vi "Request Multiple Frames.vi"(8 "error in (no error)":errorcluster, 10 "Requests":T1[](array[typedef]), 11 "connection info":T2) -> (0 "error out":errorcluster, 2 "Response Frames":T4[](array[typedef]) {"payload" format="%x"; "timestamp" format="%<%.7X\n%x>T"; "type" items=["CAN Data"=0, "CAN Remote"=1, "CAN Bus Error"=2, "CAN 2.0 Data"=8, "CAN FD Data"=16, "CAN FD+BRS Data"=24, "J1939 Data"=192, "Delay"=224, "Log Trigger"=225, "Start Trigger"=226]; "identifier" format="%x"}, 3 "connection info":T2)   [LabVIEW 2019, in "J1939 Addon Shared.lvlib"]
uses:
  J1939 Addon Shared.lvlib
  <vilib>/xnet/xnet.llb/XNET Frame CAN.ctl
  <vilib>/xnet/xnet.llb/XNET Frame Type CAN.ctl
  <vilib>/NI/STM/TCP/TCP Connection Info.ctl
  <vilib>/NI/STM/SubVIs/MetaDataElement.ctl
  Types/Request Message.ctl
  <vilib>/NI/NI VeriStand Addon Network Comm/Shared/NI VeriStand Addon Network Comm Shared.lvlib
  <vilib>/NI/STM/NI STM.lvlib
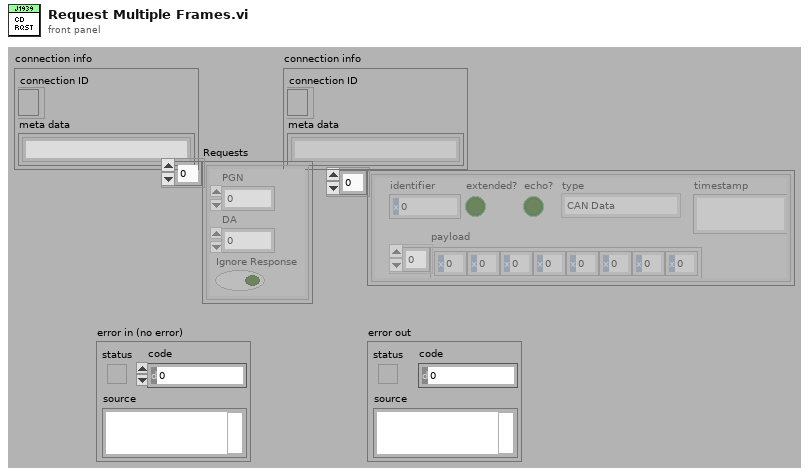
[diagram p1: front panel]
types:
  T1 = typedef "J1939 Addon Shared.lvlib/Request Message.ctl" = cluster{"PGN":u32, "DA":u8, "Ignore Response":bool}
  T2 = typedef "NI STM.lvlib/TCP Connection Info.ctl" = cluster{"connection ID":refnum<k5>, "meta data":T3[]}
  T3 = typedef "NI STM.lvlib/MetaDataElement.ctl" = string
  T4 = typedef "XNET Frame CAN.ctl" = cluster{"timestamp":timestamp, "payload":u8[], "identifier":u32, "type":T5, "extended?":bool, "echo?":bool}
  T5 = typedef "XNET Frame Type CAN.ctl" = u8
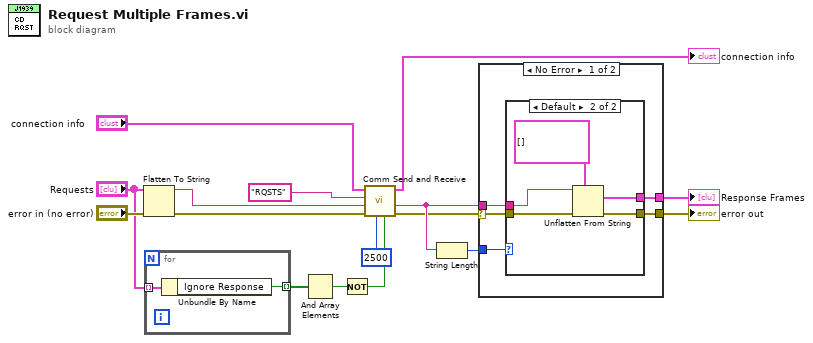
[diagram p0: block diagram]
diagram:
  n1 = Flatten To String(anything="Requests", error in (no error)="error in (no error)") -> (data string=w5:string, error out=w16:errorcluster)  [unwired: 2 in, 1 out]
  n2 = for {
    tunnel: "Requests" -> [w18] mode=indexing
    tunnel: [w17] -> w3 mode=indexing
    n3 = Unbundle By Name(w18) -> ("Ignore Response"=w17:bool)
  }
  n4 = And Array Elements(Boolean array=w3) -> (logical AND=w2:bool)
  n5 = Not(x=w2) -> (.not. x?=w1:bool)
  n6 = call <vilib>:"Comm Send and Receive.vi"("Resp Required?"=w1, "Timeout (ms)"=u32 2500 ("Timeout ms (5000)"), "error in (no error)"=w16, "Data"=w5, "Name"="RQSTS" ("Command"), "connection info"="connection info") -> ("error out"=w11:errorcluster, "Data"=w12:string, "connection info"=→"connection info":T2)  [unwired: 2 in, 1 out]
  n7 = String Length(string=w12) -> (length=w13:i32)
  n8 = case shown="No Error" w11 {
    selector: w11 -> [w20 w30]
    tunnel: [w23 w30] -> w7
    tunnel: w13 -> [w22 _]
    tunnel: w12 -> [w21 _]
    tunnel: [w19 _] -> w10
    frame No Error {
      n9 = case shown="Default" w22 {
        tunnel: w20 -> [w24 w29]
        tunnel: w21 -> [_ w25]
        tunnel: [w24 w28] -> w23
        tunnel: [_ w27] -> w19
        frame 0 {
        }
        frame Default {
          n10 = Unflatten From String(type=T4[] [], binary string=w25, error in (no error)=w29) -> (value=w27:T4[], error out=w28:errorcluster)  [unwired: 2 in, 1 out]
        }
      }
    }
    frame Error {
    }
  }
  "Response Frames" <- w10
  "error out" <- w7
